vi "Destruct.vi"(7 "Destroy Data Block? (t)":bool=TRUE, 8 "error in (no error)":errorcluster, 11 "PLC in":refnum<class "MB PLC Client.lvclass">) -> (0 "error out":errorcluster)   [LabVIEW 2018, in "MB PLC Client.lvlib" / "MB PLC Client.lvclass"]
uses:
  MB PLC Client.lvclass
  MB PLC Client.lvclass/MB PLC Client.ctl
  <vilib>/Plasmionique/MB Master/MB_Master/MB_Master.lvclass
  Data/MB Data Block.lvclass
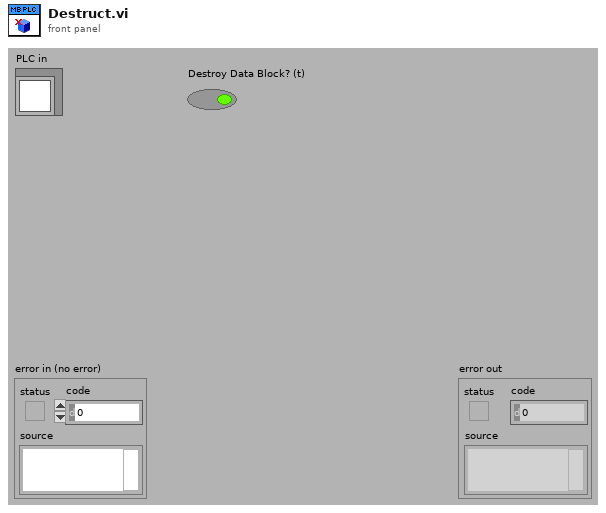
[diagram p1: front panel]
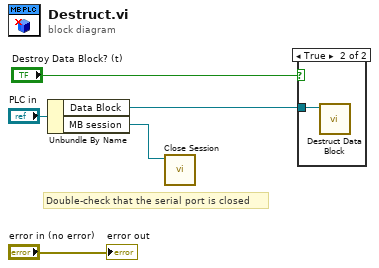
[diagram p0: block diagram]
diagram:
  # "Double-check that the serial port is closed"
  n1 = Unbundle By Name("PLC in") -> ("Data Block"=w1:refnum<data-value>, "MB session"=w3:refnum<class "MB_Master.lvclass">)
  n2 = call-dynamic "Close Session.vi"("MB session in"=w3) -> ()  [unwired: 10 in, 1 out]
  n3 = case shown="True" "Destroy Data Block? (t)" {
    tunnel: w1 -> [_ w6]
    frame False {
    }
    frame True {
      n4 = call "Destruct Data Block.vi"("Cache Ref in"=w6) -> ()  [unwired: 10 in, 1 out]
    }
  }
  "error out" <- "error in (no error)"
